vi "Rotation3d_GetQuaterion.vi"(11 "in Rotation3d":T2={"Q_quaternion"={"R"=1.0, "V"=[0.0, 0.0, 0.0]}}) -> (3 "out Quaterion":T1={"R"=1.0, "V"=[0.0, 0.0, 0.0]})   [LabVIEW 2019, in "Trajectory_Library.lvlib"]
doc: "Returns the quaternion representation of the Rotation3d.\n\nParameters:\n - in ROTATION3D - This ROTATION3D data structure\n\nReturns:\n - out Quaternion -- The quaternion representation of the Rotation3d."
uses:
  Trajectory_Library.lvlib
  ROTATION3D.ctl
  QUATERNION.ctl
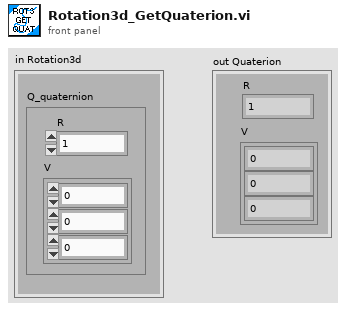
[diagram p1: front panel]
types:
  T1 = typedef "Trajectory_Library.lvlib/QUATERNION.ctl" = cluster{"R":dbl, "V":dbl[]}
  T2 = typedef "Trajectory_Library.lvlib/ROTATION3D.ctl" = cluster{"Q_quaternion":T1}
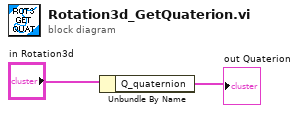
[diagram p0: block diagram]
diagram:
  n1 = Unbundle By Name("in Rotation3d") -> ("Q_quaternion"=→"out Quaterion":T1)
